vi "zmq_poll_scalar.vi"(4 "error in":errorcluster, 5 "timeout":i32=100, 6 "poll type":T1=enum."In/Out", 7 "sockets":refnum<class "zmq_socket.lvclass">[](array[class])) -> (0 "error out":errorcluster, 1 "timed out?":bool, 2 "nevents":i32, 3 "polled events":T1[](array[typedef]))   [LabVIEW 2010, in "zeromq.lvlib" / "zmq_socket.lvclass"]
doc: "Poll multiple sockets and for events. Blocks for <b>timeout</b> milliseconds or until an event occur on any of the given <b>sockets</b>. If no event happens, then <b>timed out?</b> is True.\n\n<b>poll type</b> contains the events to look for, and is applied to every socket given. If not specified, sockets are polled for all events.\n\nIf <b>timeout</b> is zero, the function returns immediately, regardless of whether any events are waiting. If <b>timeout</b> is negative, the function will block until an event occurs.\n\nDetailed API documentation: http://api.zeromq.org/3-2:zmq-polls"
uses:
  zmq_socket.lvclass
  poll_type.ctl
  zeromq.lvlib
panel:
  # "ØMQ"
  # "labview"
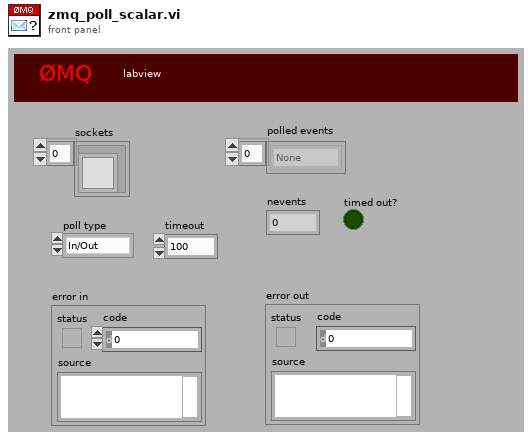
[diagram p1: front panel]
types:
  T1 = typedef "zeromq.lvlib/poll_type.ctl" = enum16{"None", "In", "Out", "In/Out"}
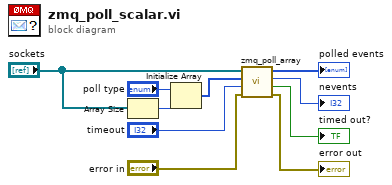
[diagram p0: block diagram]
diagram:
  n1 = Array Size(array="sockets") -> (size(s)=w10:i32)
  n2 = Initialize Array("poll type", w10) -> (w6:T1[])
  n3 = call "zmq_poll_array.vi"("error in"="error in", "timeout"="timeout", "poll type"=w6, "sockets"="sockets") -> ("error out"=→"error out":errorcluster, "timed out?"=→"timed out?":bool, "nevents"=→"nevents":i32, "polled events"=→"polled events":T1[])
